vi "Ultrasonic_Get_Range.vi"(3 "error in (no error)":errorcluster, 5 "SonarMB1010DigitalDevRef":T1={"CounterDevRef"={"DevStatus"={"status"=FALSE, "code"=0, "source"=""}, "CntIndex"=enum."Invalid"}, "Scaling factor (s/in)"=0.0}) -> (0 "error out":errorcluster, 1 "Range":dbl, 2 "SonarMB1010DigitalDevRef 2":T1={"CounterDevRef"={"DevStatus"={"status"=FALSE, "code"=0, "source"=""}, "CntIndex"=enum."Invalid"}, "Scaling factor (s/in)"=0.0})   [LabVIEW 2017, in "ArgosLib.lvlib"]
uses:
  ArgosLib.lvlib
  <vilib>/Rock Robotics/WPI/Ultrasonic/WPI_SonarMB1010DigitalDeviceRef.ctl
  <vilib>/Rock Robotics/WPI/Counter/WPI_CounterDevRef.ctl
  <vilib>/Rock Robotics/SystemInterfaces/Counter/FPGA_CounterCtrSystemIndex.ctl
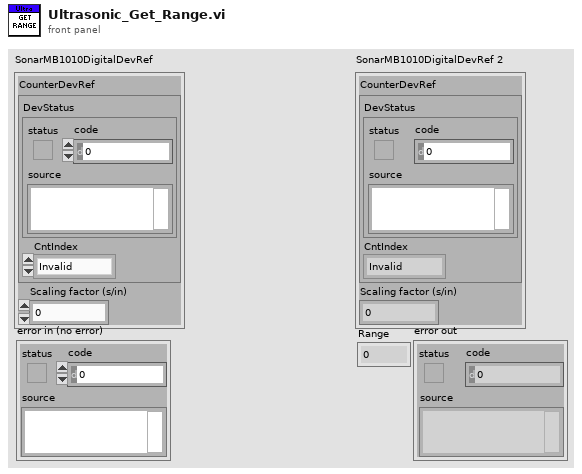
[diagram p1: front panel]
types:
  T1 = typedef "WPI_SonarMB1010DigitalDeviceRef.ctl" = cluster{"CounterDevRef":T2, "Scaling factor (s/in)":dbl}
  T2 = typedef "WPI_CounterDevRef.ctl" = cluster{"DevStatus":errorcluster, "CntIndex":T3}
  T3 = typedef "FPGA_CounterCtrSystemIndex.ctl" = enum8{"Ctr 0", "Ctr 1", "Ctr 2", "Ctr 3", "Ctr 4", "Ctr 5", "Ctr 6", "Ctr 7", "Invalid"}
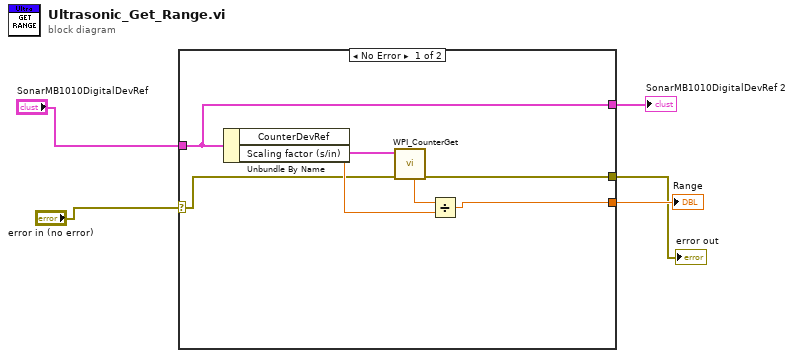
[diagram p0: block diagram]
diagram:
  n1 = case shown="No Error" "error in (no error)" {
    selector: "error in (no error)" -> [w8 w13]
    tunnel: "SonarMB1010DigitalDevRef" -> [w7 w14]
    tunnel: [w9 _] -> w4
    tunnel: [w7 w14] -> w2
    tunnel: [w6 w13] -> w1
    frame No Error {
      n2 = Unbundle By Name(w7) -> ("CounterDevRef"=w12:T2, "Scaling factor (s/in)"=w10:dbl)
      n3 = call <vilib>:"WPI_CounterGet.vi"("error in (no error)"=w8, "CounterDevRef in"=w12) -> ("error out"=w6:errorcluster, "Period (sec)"=w11:dbl)  [unwired: 4 in, 4 out]
      n4 = Divide(x=w11, y=w10) -> (x/y=w9:dbl)
    }
    frame Error {
    }
  }
  "SonarMB1010DigitalDevRef 2" <- w2
  "Range" <- w4
  "error out" <- w1
